vi "Ctor.vi"(8 "error in (no error)":errorcluster) -> (0 "error out":errorcluster, 3 "SB App out":refnum<class "SB App.lvclass">)   [LabVIEW 2020, in "SB App.lvlib" / "SB App.lvclass"]
uses:
  SB App.lvclass
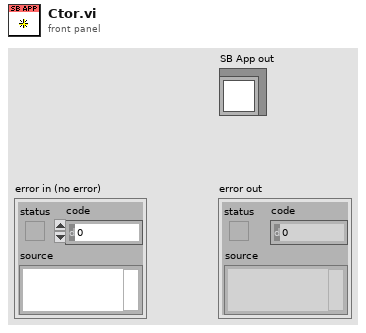
[diagram p1: front panel]
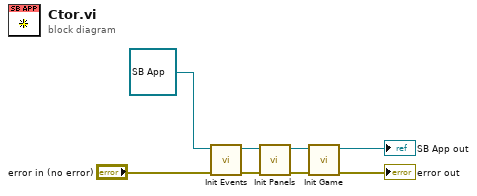
[diagram p0: block diagram]
diagram:
  n1 = call "Init Events.vi"("error in (no error)"="error in (no error)", "SB App in"=refnum<class "SB App.lvclass"> refnum) -> ("error out"=w5:errorcluster, "SB App out"=w6:refnum<class "SB App.lvclass">)  [unwired: 8 in]
  n2 = call "Init Panels.vi"("error in (no error)"=w5, "SB App in"=w6) -> ("error out"=w3:errorcluster, "SB App out"=w4:refnum<class "SB App.lvclass">)  [unwired: 8 in]
  n3 = call "Init Game.vi"("error in (no error)"=w3, "SB App in"=w4) -> ("error out"=→"error out":errorcluster, "SB App out"=→"SB App out":refnum<class "SB App.lvclass">)  [unwired: 8 in]
